vi "niDTS BT Tx Test Get Default Limits.vi"(0 "Dummy Test Handle in":T9, 11 "error in (no error)":errorcluster) -> (4 "Dummy Test Handle out":T9, 6 "Default USL":T1 {"OBW Resutls"."Stop Frequency (Hz)" format="%#_4p"; "OBW Resutls"."Start Frequency (Hz)" format="%#_4p"}, 8 "Default LSL":T1 {"OBW Resutls"."Stop Frequency (Hz)" format="%#_4p"; "OBW Resutls"."Start Frequency (Hz)" format="%#_4p"}, 15 "error out":errorcluster)   [LabVIEW 2014, in "niDTS BT.lvlib"]
uses:
  niDTS BT.lvlib
  Includes/niDTS BT Tx Test INC Handle.ctl
  Objects/BASE_class/niDTS BT Tx Test.lvclass
  Includes/niDTS BT Tx Test INC Results.ctl
  Includes/niDTS BT Tx Test INC IBE Results.ctl
  Includes/niDTS BT Tx Test INC OBW Results.ctl
  Includes/niDTS BT Tx Test INC TXP Results.ctl
  Includes/niDTS BT Tx Test INC DEVM Results.ctl
  Includes/niDTS BT Tx Test INC CF Stability Results.ctl
  Includes/niDTS BT Tx Test INC CFO Resutls.ctl
  Includes/niDTS BT Tx Test INC Character Results.ctl
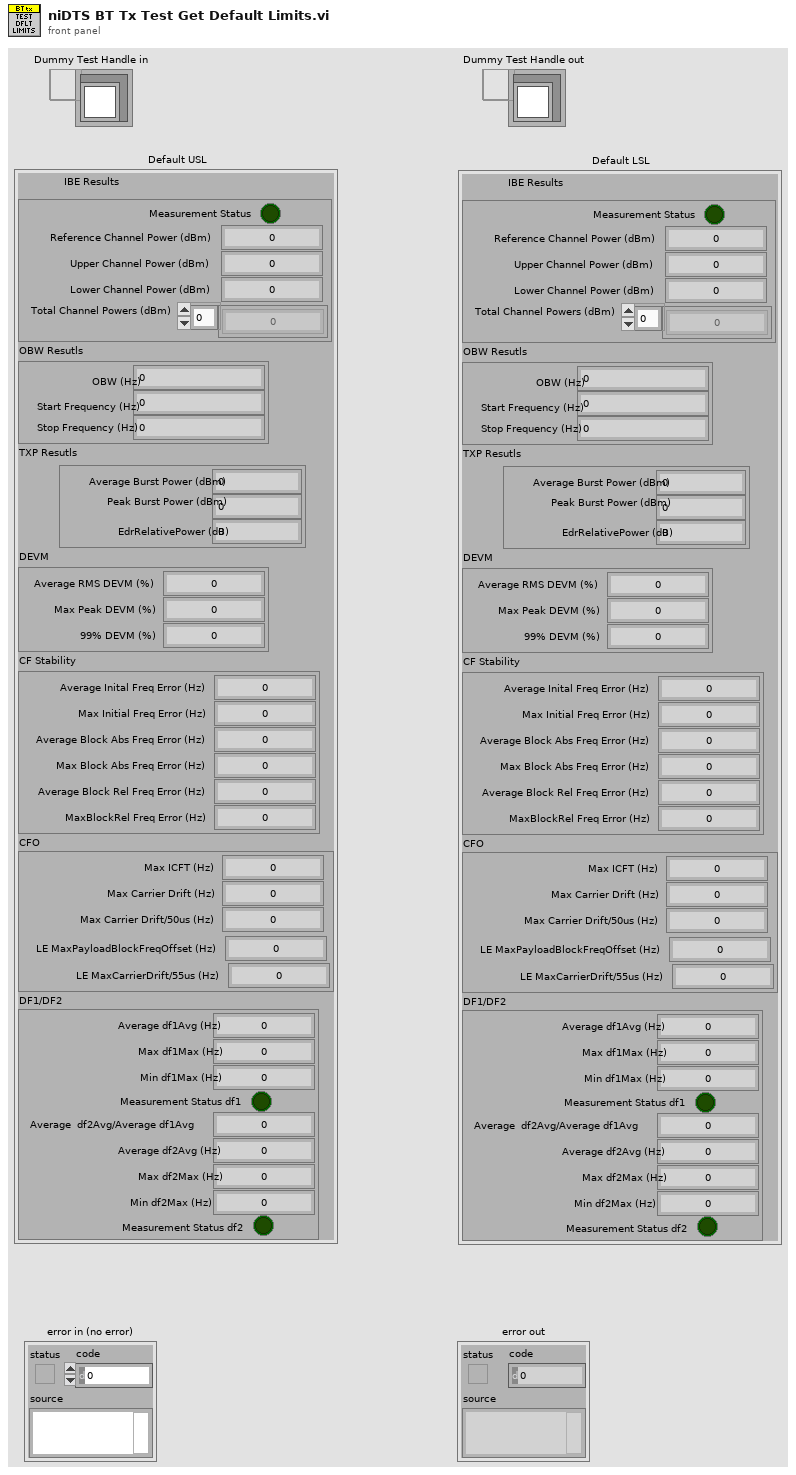
[diagram p1: front panel]
types:
  T1 = typedef "niDTS BT.lvlib/niDTS BT Tx Test INC Results.ctl" = cluster{"IBE Results":T2, "OBW Resutls":T3, "TXP Resutls":T4, "DEVM":T5, "CF Stability":T6, "CFO":T7, "DF1/DF2":T8}
  T2 = typedef "niDTS BT.lvlib/niDTS BT Tx Test INC IBE Results.ctl" = cluster{"Measurement Status":bool, "Reference Channel Power (dBm)":dbl, "Upper Channel Power (dBm)":dbl, "Lower Channel Power (dBm)":dbl, "Total Channel Powers (dBm)":dbl[]}
  T3 = typedef "niDTS BT.lvlib/niDTS BT Tx Test INC OBW Results.ctl" = cluster{"OBW (Hz)":dbl, "Start Frequency (Hz)":dbl, "Stop Frequency (Hz)":dbl}
  T4 = typedef "niDTS BT.lvlib/niDTS BT Tx Test INC TXP Results.ctl" = cluster{"Average Burst Power (dBm)":dbl, "Peak Burst Power (dBm)":dbl, "EdrRelativePower (dB)":dbl}
  T5 = typedef "niDTS BT.lvlib/niDTS BT Tx Test INC DEVM Results.ctl" = cluster{"Average RMS DEVM (%)":dbl, "Max Peak DEVM (%)":dbl, "99% DEVM (%)":dbl}
  T6 = typedef "niDTS BT.lvlib/niDTS BT Tx Test INC CF Stability Results.ctl" = cluster{"Average Inital Freq Error (Hz)":dbl, "Max Initial Freq Error (Hz)":dbl, "Average Block Abs Freq Error (Hz)":dbl, "Max Block Abs Freq Error (Hz)":dbl, "Average Block Rel Freq Error (Hz)":dbl, "MaxBlockRel Freq Error (Hz)":dbl}
  T7 = typedef "niDTS BT.lvlib/niDTS BT Tx Test INC CFO Resutls.ctl" = cluster{"Max ICFT (Hz)":dbl, "Max Carrier Drift (Hz)":dbl, "Max Carrier Drift/50us (Hz)":dbl, "LE MaxPayloadBlockFreqOffset (Hz)":dbl, "LE MaxCarrierDrift/55us (Hz)":dbl}
  T8 = typedef "niDTS BT.lvlib/niDTS BT Tx Test INC Character Results.ctl" = cluster{"Average df1Avg (Hz)":dbl, "Max df1Max (Hz)":dbl, "Min df1Max (Hz)":dbl, "Measurement Status df1":bool, "Average  df2Avg/Average df1Avg":dbl, "Average df2Avg (Hz)":dbl, "Max df2Max (Hz)":dbl, "Min df2Max (Hz)":dbl, "Measurement Status df2":bool}
  T9 = typedef "niDTS BT.lvlib/niDTS BT Tx Test INC Handle.ctl" = refnum<data-value>
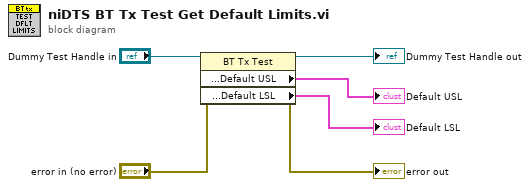
[diagram p0: block diagram]
diagram:
  n1 = property class="BT Tx Test"(reference="Dummy Test Handle in", error in="error in (no error)") -> (reference out=→"Dummy Test Handle out":T9, error out=→"error out":errorcluster, "Properties:Default Limits:Default USL"=→"Default USL":T1, "Properties:Default Limits:Default LSL"=→"Default LSL":T1)
